vi "TDT-Get Device Properties.vi"(0 "TDT-Device Config":T1, 7 "App Prefix":string, 11 "error in (no error)":errorcluster, 12 "Biosemi":bool) -> (4 "Circuit File":string, 6 "Num Outputs":i32, 8 "Num Inputs":i32, 10 "Tag":string, 14 "Gain":dbl=nan, 15 "error out":errorcluster)   [LabVIEW 2020]
uses:
  Typedefs/TDT-Device Config.ctl
  Typedefs/TDT-Output source.ctl
  Typedefs/TDT-Device ID.ctl
  Typedefs/TDT-Input source.ctl
  0f9ec20f-2efd-46df-9665-33f75441c04e.vi
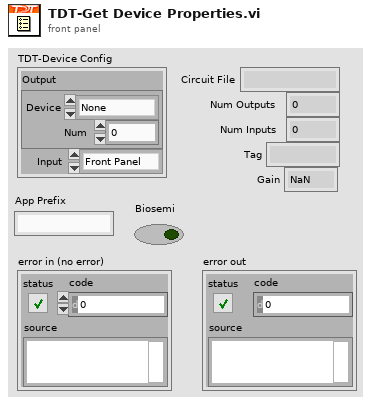
[diagram p1: front panel]
types:
  T1 = typedef "TDT-Device Config.ctl" = cluster{"Output":T2, "Input":T4}
  T2 = typedef "TDT-Output source.ctl" = cluster{"Device":T3, "Num":i32}
  T3 = typedef "TDT-Device ID.ctl" = enum16{"None", "PA5", "RP2", "RL2", "RA16", "RV8", "RX5", "RX6", "RX7", "RX8", "RZ2", "RZ5", "RZ6"}
  T4 = typedef "TDT-Input source.ctl" = enum16{"Front Panel", "RA4LI", "RA16LI"}
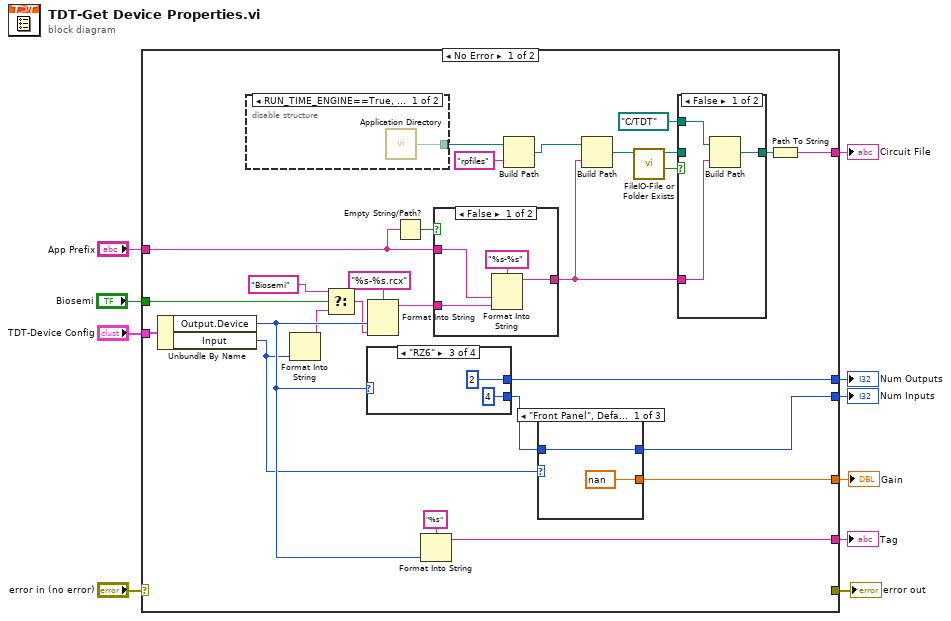
[diagram p0: block diagram]
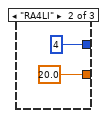
[diagram p4: hidden frame]
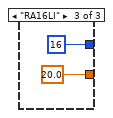
[diagram p5: hidden frame]
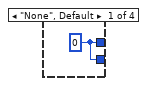
[diagram p6: hidden frame]
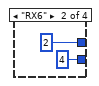
[diagram p7: hidden frame]
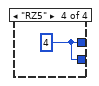
[diagram p8: hidden frame]
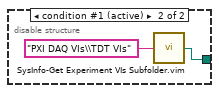
[diagram p9: hidden frame]
diagram:
  n1 = case shown="No Error" "error in (no error)" {
    selector: "error in (no error)" -> [_ w62]
    tunnel: "TDT-Device Config" -> [w37 _]
    tunnel: [w18 _] -> w8
    tunnel: [w30 _] -> w6
    tunnel: [w33 _] -> w7
    tunnel: [_ w62] -> w5
    tunnel: [w32 _] -> w4
    tunnel: [w29 _] -> w3
    tunnel: "App Prefix" -> [w25 _]
    tunnel: "Biosemi" -> [w22 _]
    frame No Error {
      n2 = Unbundle By Name(w37) -> ("Output.Device"=w34:T3, "Input"=w23:T4)
      n3 = disable-structure shown="RUN_TIME_ENGINE==True, Default" {
        disable-tunnel: [w59 w61] -> w28
        frame condition #0 {
          n4 = call <vilib>:"Application Directory.vi"() -> ("Application Directory"=w59:path)
        }
        frame condition #1 (active) {
          n5 = call "SysInfo-Get Experiment VIs Subfolder.vim"("subfolder"="PXI DAQ VIs\\TDT VIs") -> ("full path"=w61:path)  [unwired: 4 in]
        }
      }
      n6 = Format Into String(w23) -> (resulting string=w20:string)  [unwired: 3 in, 1 out]
      n7 = Select(t="Biosemi", s=w22, f=w20) -> (s? t:f=w19:string)
      n8 = case shown="\"RZ6\"" w34 {
        tunnel: [w53 2 2 w58] -> w33
        tunnel: [w53 4 4 w58] -> w31
        frame "None", Default {
          w53 = 0
        }
        frame "RX6" {
        }
        frame "RZ6" {
        }
        frame "RZ5" {
          w58 = 4
        }
      }
      n9 = Format Into String(format string="%s-%s.rcx", w34, w19) -> (resulting string=w17:string)  [unwired: 2 in, 1 out]
      n10 = Empty String/Path?(string/path=w25) -> (empty?=w24:bool)
      n11 = Format Into String(format string="%s", w34) -> (resulting string=w32:string)  [unwired: 2 in, 1 out]
      n12 = case shown="False" w24 {
        tunnel: w17 -> [w44 w46]
        tunnel: w25 -> [w43 _]
        tunnel: [w42 w46] -> w12
        frame False {
          n13 = Format Into String(format string="%s-%s", w43, w44) -> (resulting string=w42:string)  [unwired: 2 in, 1 out]
        }
        frame True {
        }
      }
      n14 = Build Path(base path=w28, name or relative path="rpfiles") -> (appended path=w26:path)
      n15 = case shown="\"Front Panel\", Default" w23 {
        tunnel: w31 -> [w48 _ _]
        tunnel: [w48 4 16] -> w30
        tunnel: [nan 20.0 20.0] -> w29
        frame "Front Panel", Default {
        }
        frame "RA4LI" {
        }
        frame "RA16LI" {
        }
      }
      n16 = Build Path(base path=w26, name or relative path=w12) -> (appended path=w16:path)
      n17 = call "FileIO-File or Folder Exists.vi"("path"=w16) -> ("Exists?"=w14:bool, "dup path"=w15:path)  [unwired: 7 in, 2 out]
      n18 = case shown="False" w14 {
        tunnel: w15 -> [_ w41]
        tunnel: [w39 w41] -> w13
        tunnel: w12 -> [w40 _]
        tunnel: path "C:/TDT" -> [w38 _]
        frame False {
          n19 = Build Path(base path=w38, name or relative path=w40) -> (appended path=w39:path)
        }
        frame True {
        }
      }
      n20 = Path To String(path=w13) -> (string=w18:string)
    }
    frame Error {
    }
  }
  "error out" <- w5
  "Circuit File" <- w8
  "Num Outputs" <- w7
  "Num Inputs" <- w6
  "Tag" <- w4
  "Gain" <- w3
